vi "SerialPortInit960.vi"(8 "错误输入":errorcluster caption="错误输入（无错误）", 11 "COMIn":refnum<visa-resource-name>="COM1") -> (0 "错误输出":errorcluster, 3 "COMOut":refnum<visa-resource-name>)   [LabVIEW 2013]
uses:
  <vilib>/Instr/_visa.llb/VISA Flush IO Buffer Mask.ctl
  <vilib>/Instr/_visa.llb/VISA Configure Serial Port (Instr).vi
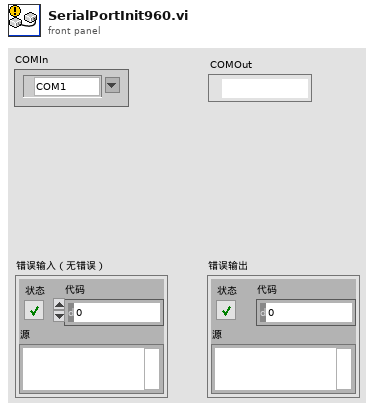
[diagram p1: front panel]
types:
  T1 = cluster{"波特率":u32, "数据比特":u16, "奇偶":enum16{"None", "Odd", "Even", "Mark", "Space"}, "停止位":u16, "流控制":u16}
  T2 = typedef "VISA Flush IO Buffer Mask.ctl" = u16
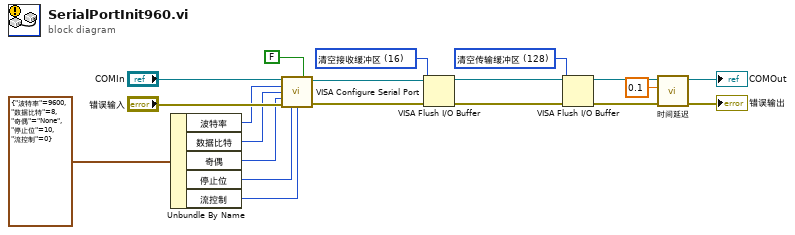
[diagram p0: block diagram]
diagram:
  w3 = T2 128 items=["清空接收缓冲区"=16, "向设备写入传输缓冲区"=32, "清空接收缓冲区（无I/O）"=64, "清空传输缓冲区"=128] ("Mask")
  w6 = T2 16 items=["清空接收缓冲区"=16, "向设备写入传输缓冲区"=32, "清空接收缓冲区（无I/O）"=64, "清空传输缓冲区"=128] ("Mask")
  n1 = Unbundle By Name(T1 {"波特率"=9600, "数据比特"=8, "奇偶"=enum."None", "停止位"=10, "流控制"=0} ("串口设置")) -> ("波特率"=w11:u32, "数据比特"=w12:u16, "奇偶"=w13:enum16{"None", "Odd", "Even", "Mark", "Space"}, "停止位"=w14:u16, "流控制"=w9:u16)
  n2 = call-poly "VISA Configure Serial Port"("VISA resource name"="COMIn", "Enable Termination\nChar (T)"=FALSE ("Enable Termination\nChar (T)"), "baud rate (9600)"=w11, "data bits (8)"=w12, "parity (0:none)"=w13, "error in (no error)"="错误输入", "stop bits (10: 1 bit)"=w14, "flow control (0:none)"=w9) -> ("VISA resource name out"=w7:refnum<visa-resource-name>, "error out"=w8:errorcluster)  [unwired: 2 in, 4 out]
  n3 = VISA Flush I/O Buffer(VISA resource name=w7, mask (16)=w6, error in (no error)=w8) -> (VISA resource name out=w4:refnum<visa-resource-name>, error out=w5:errorcluster)
  n4 = VISA Flush I/O Buffer(VISA resource name=w4, mask (16)=w3, error in (no error)=w5) -> (VISA resource name out=→"COMOut":refnum<visa-resource-name>, error out=w15:errorcluster)
  n5 = call "时间延迟"("error in (no error)"=w15, "Delay Time (s)"=0.1) -> ("error out"=→"错误输出":errorcluster)  [unwired: 9 in]
